vi "Main.vi"() -> ()   [LabVIEW 2017, in "Application.lvlib"]
doc: "This VI is the main application VI in the Delacor QMH project template. This application VI is implemented as a simple state machine, which communicates with two different Delacor QMH modules.\n_____\nBased on Delacor QMH Project Template 3.1.0.34."
uses:
  Application.lvlib
  Application Data--cluster.ctl
  State--enum.ctl
  GUI/GUI.lvlib
  Konfiguracja/Konfiguracja.lvlib
  Akwizycja/Akwizycja.lvlib
panel:
  in  "Debug":bool
  in  "Start Akwizycja Module":bool
  in  "Stop Akwizycja Module":bool caption="Start Akwizycja Module"
  out "Akwizycja Running?":bool
  out "version":string
  in  "Hide GUI Module":bool
  in  "Show GUI Module":bool
  in  "Stop GUI Module":bool
  in  "Start GUI Module":bool caption="Start Akwizycja Module"
  out "GUI Running?":bool
  in  "Hide Konfiguracja Module":bool
  in  "Show Konfiguracja Module":bool
  in  "Stop Konfiguracja Module":bool
  in  "Start Konfiguracja Module":bool
  out "Konfiguracja Running?":bool
  out "Status":string
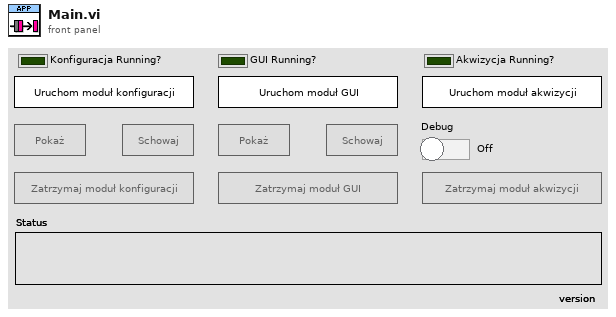
[diagram p1: front panel]
types:
  T1 = typedef "Application.lvlib/State--enum.ctl" = enum16{"Initialize", "Initialize Panel", "UI Interlocks", "Update Status", "Wait for Event", "Exit"}
  T2 = typedef "Application.lvlib/Application Data--cluster.ctl" = cluster{"Status":string, "Konfiguracja Controls":refnum<vi>[], "GUI Controls":refnum<vi>[], "Akwizycja Controls":refnum<vi>[]}
  T3 = typedef "Akwizycja.lvlib/Broadcast Events--cluster.ctl" = cluster{"Module Did Init":refnum<user-event>, "Status Updated":refnum<user-event>, "Error Reported":refnum<user-event>, "Module Did Stop":refnum<user-event>, "Update Module Execution Status":refnum<user-event>}
  T4 = typedef "GUI.lvlib/Broadcast Events--cluster.ctl" = cluster{"Module Did Init":refnum<user-event>, "Status Updated":refnum<user-event>, "Error Reported":refnum<user-event>, "Module Did Stop":refnum<user-event>, "Update Module Execution Status":refnum<user-event>, "Subpanel VI Loaded":refnum<user-event>}
  T5 = typedef "Konfiguracja.lvlib/Broadcast Events--cluster.ctl" = cluster{"Module Did Init":refnum<user-event>, "Status Updated":refnum<user-event>, "Error Reported":refnum<user-event>, "Module Did Stop":refnum<user-event>, "Update Module Execution Status":refnum<user-event>, "Subpanel VI Loaded":refnum<user-event>}
  T6 = enum8{"Enabled", "Disabled", "Disabled and Grayed Out"}
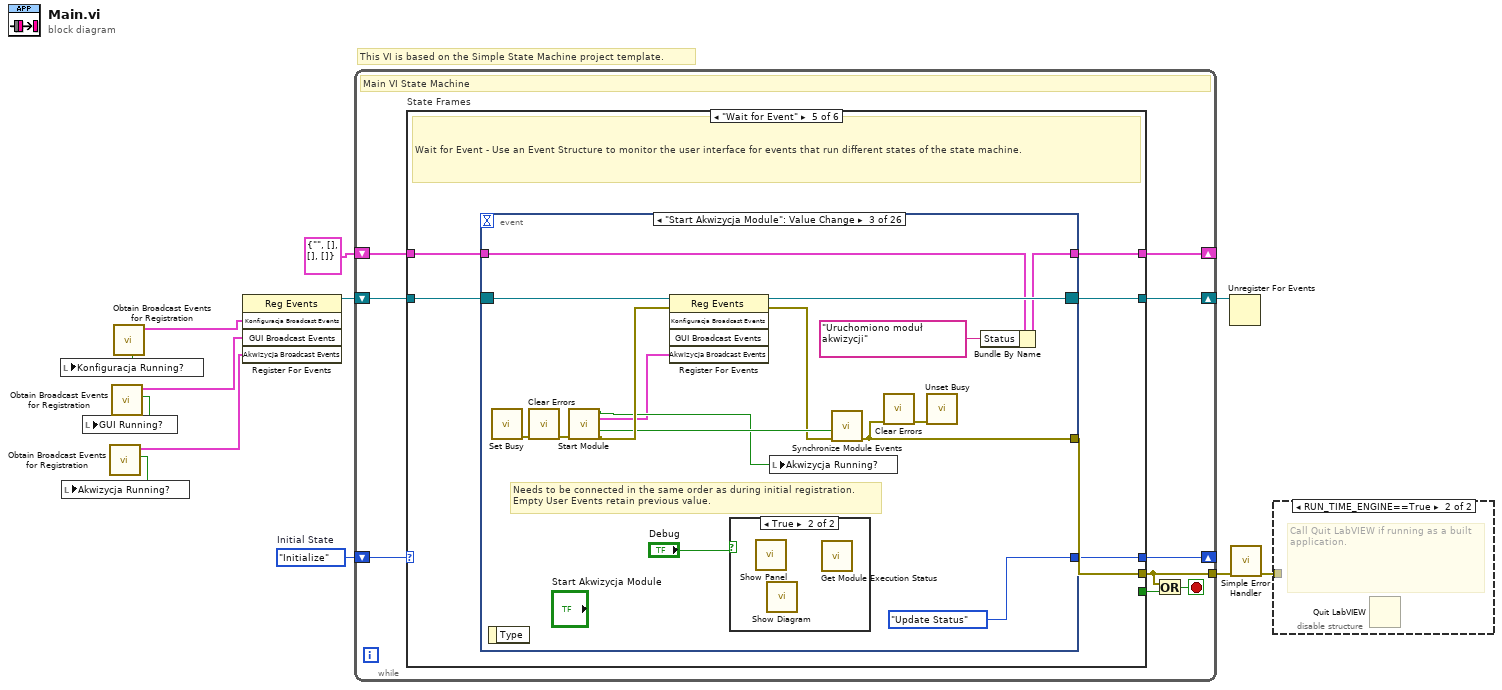
[diagram p0: block diagram]
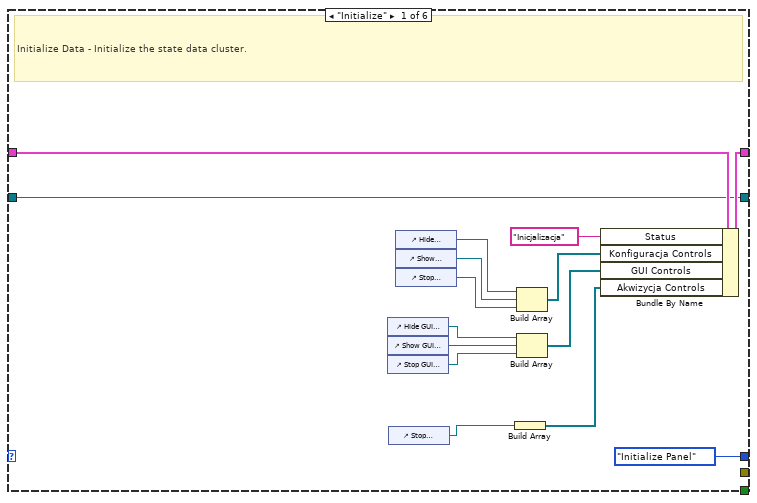
[diagram p2: hidden frame]
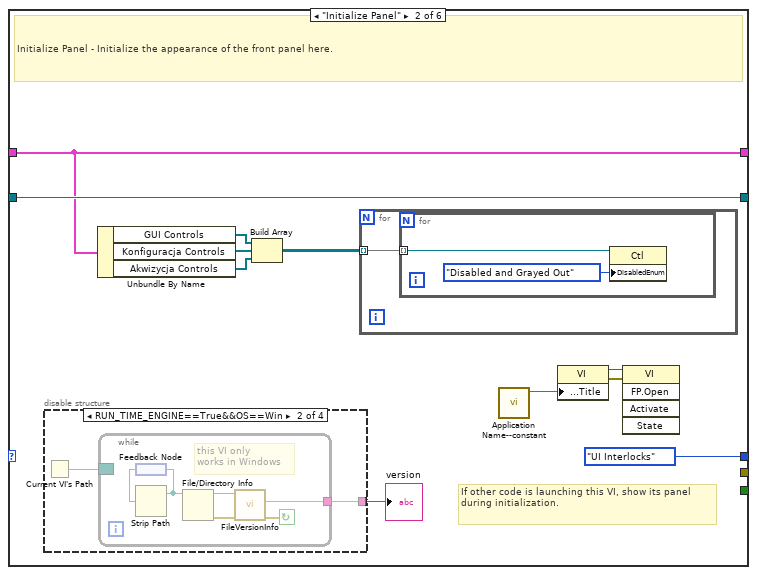
[diagram p3: hidden frame]
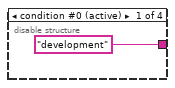
[diagram p4: hidden frame]
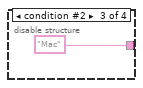
[diagram p5: hidden frame]
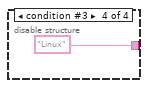
[diagram p6: hidden frame]
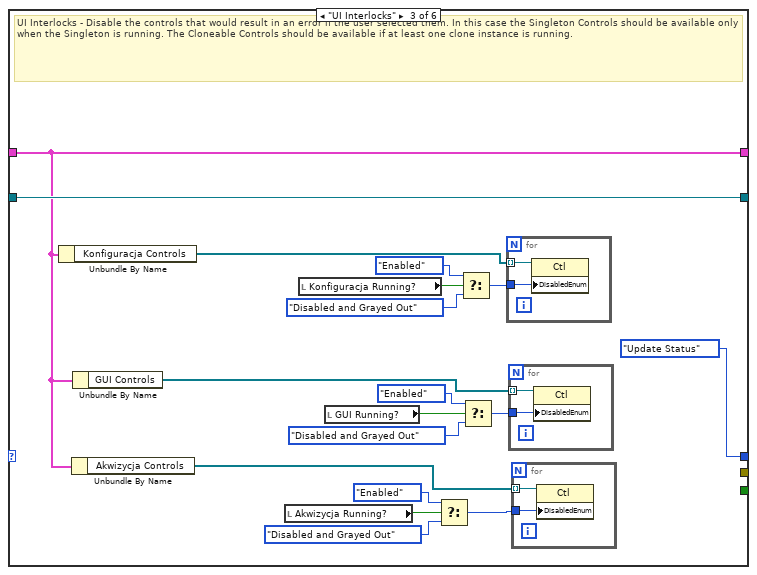
[diagram p7: hidden frame]
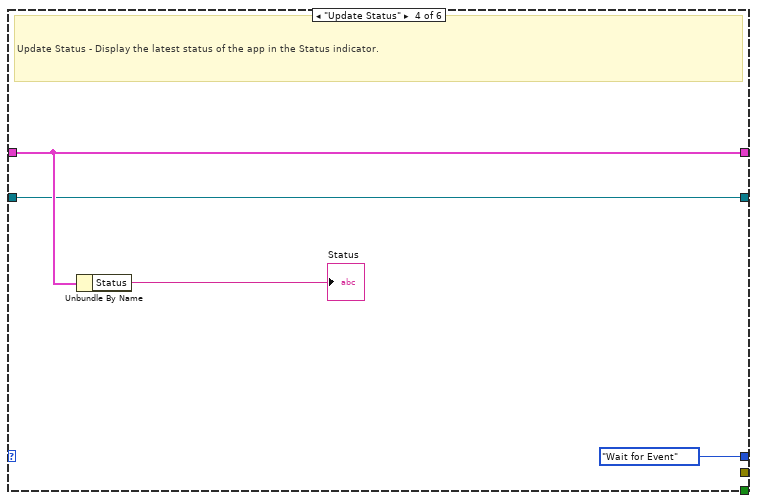
[diagram p8: hidden frame]
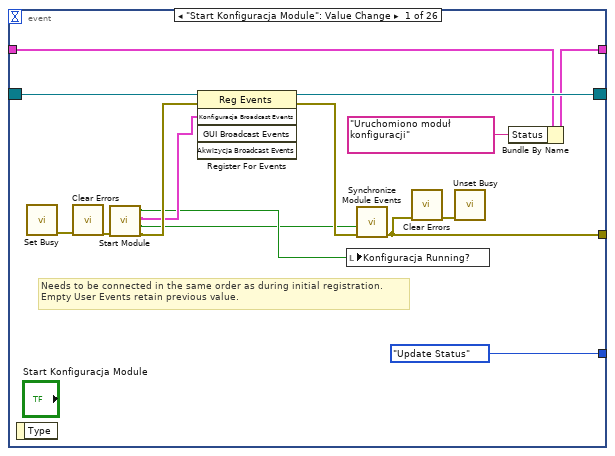
[diagram p9: hidden frame]
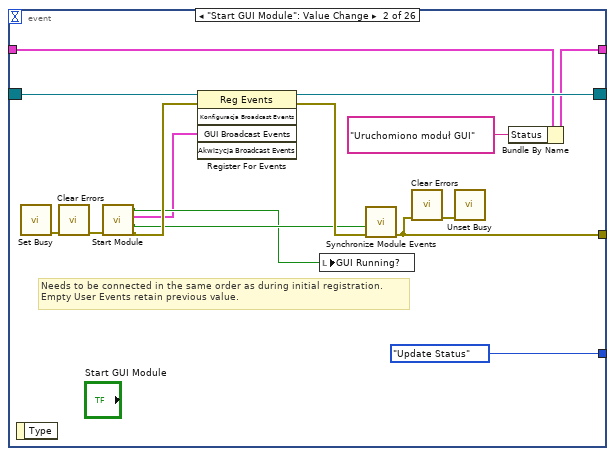
[diagram p10: hidden frame]
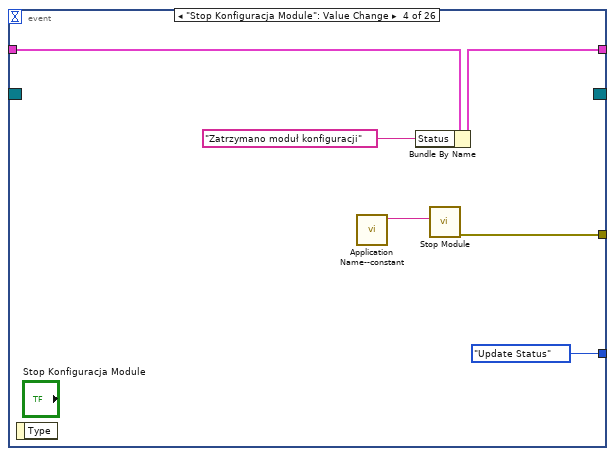
[diagram p12: hidden frame]
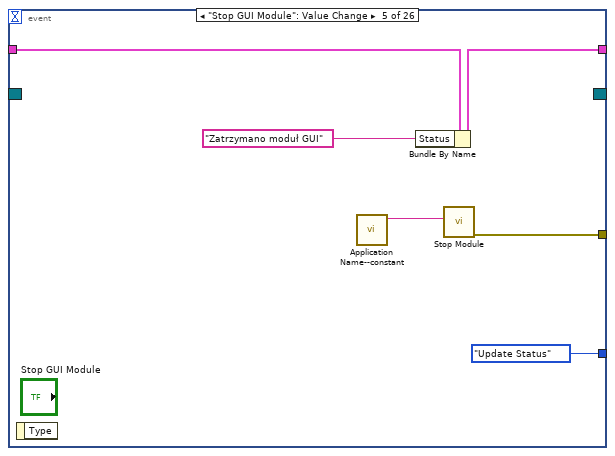
[diagram p13: hidden frame]
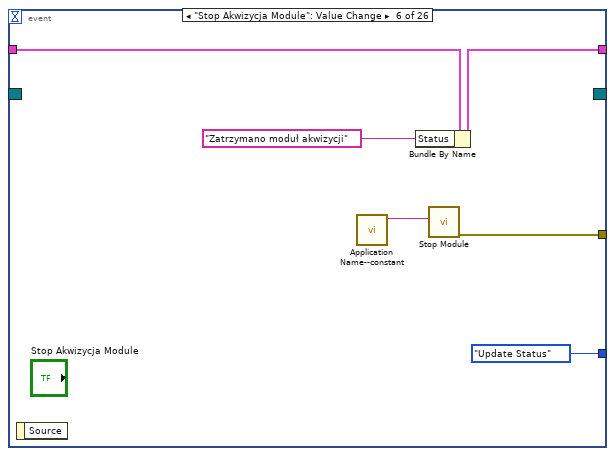
[diagram p14: hidden frame]
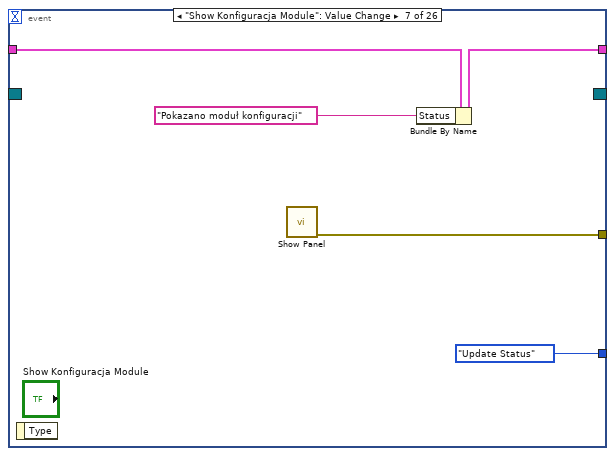
[diagram p15: hidden frame]
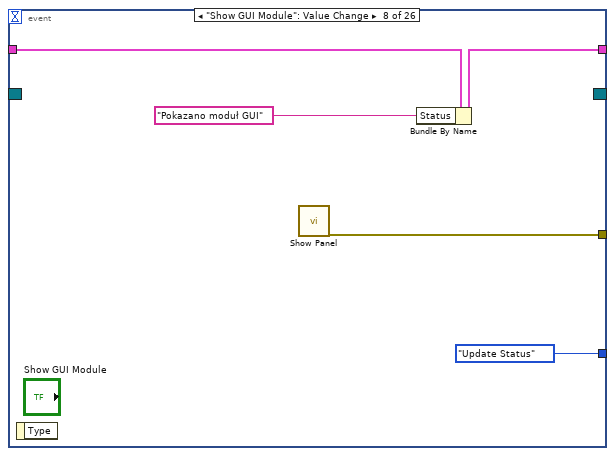
[diagram p16: hidden frame]
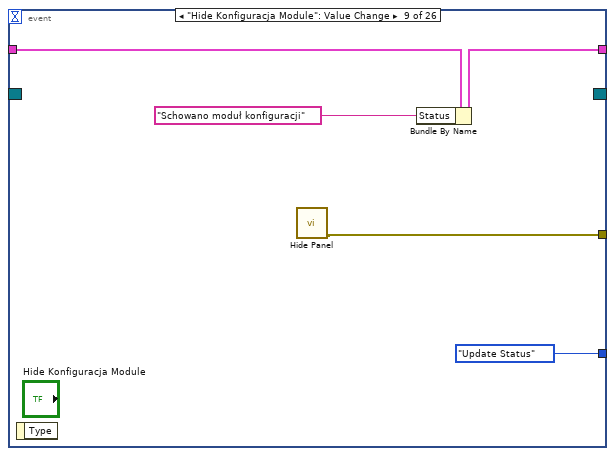
[diagram p17: hidden frame]
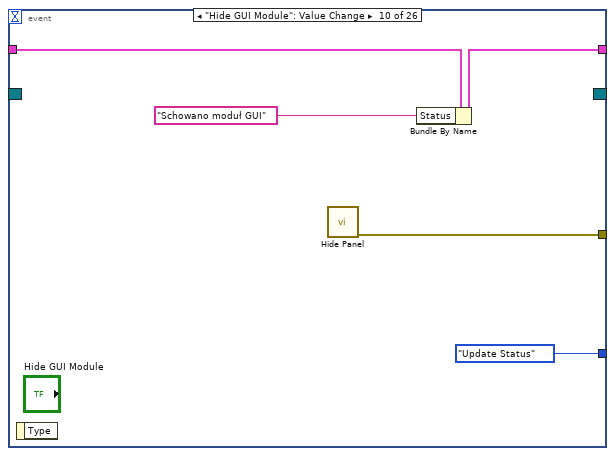
[diagram p18: hidden frame]
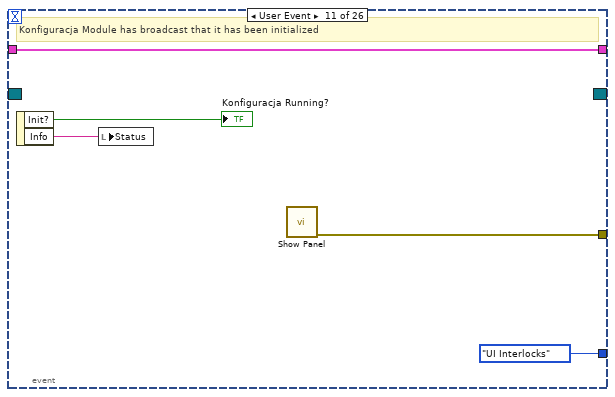
[diagram p19: hidden frame]
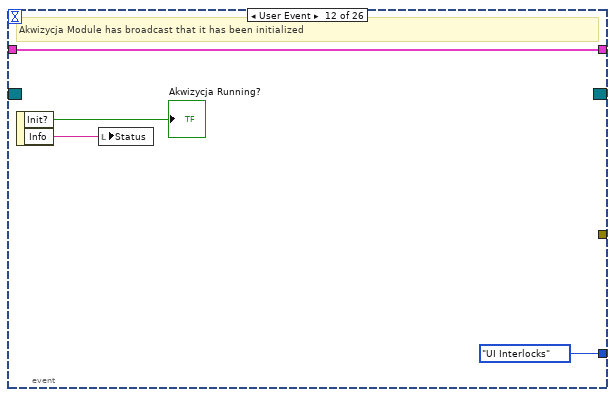
[diagram p20: hidden frame]
diagram:
  w9 = State--enum."Initialize"  # Initial State
  # "This VI is based on the Simple State Machine project template."
  n1 = call "Obtain Broadcast Events for Registration.vi"() -> ("Already running?"=w2:bool, "Akwizycja Broadcast Events"=w1:T3)  [unwired: 9 in, 1 out]
  n2 = local write "Akwizycja Running?"(w2) -> ()
  n3 = call "Obtain Broadcast Events for Registration.vi"() -> ("Already running?"=w5:bool, "GUI Broadcast Events"=w6:T4)  [unwired: 9 in, 1 out]
  n4 = local write "GUI Running?"(w5) -> ()
  n5 = call "Obtain Broadcast Events for Registration.vi"() -> ("Already running?"=w3:bool, "Konfiguracja Broadcast Events"=w4:T5)  [unwired: 9 in, 1 out]
  n6 = local write "Konfiguracja Running?"(w3) -> ()
  n7 = register-events(w4, w6, w1) -> (reference out=w8:refnum<event-registration>)  [unwired: 2 in, 1 out]
  n8 = while {
    shift-right: [w20] -> _
    shift-left: T2 {"Status"="", "Konfiguracja Controls"=[], "GUI Controls"=[], "Akwizycja Controls"=[]} ("Data Cluster") -> [w21]
    tunnel: [w16] -> w11
    shift-right: [w15] -> _
    shift-left: w9 -> [w18]
    shift-right: [w13] -> w7
    shift-left: w8 -> [w14]
    stop <- w17 stop-if-true
    # "Main VI State Machine"
    n9 = case "State Frames" shown="\"Wait for Event\"" w18 {
      tunnel: [_ _ _ _ w91 w275] -> w16
      tunnel: w21 -> [w36 w41 w67 w89 w93 w279]
      tunnel: [w35 w41 w67 w89 w92 w279] -> w20
      tunnel: [_ _ _ _ _ w278] -> w19
      tunnel: [State--enum."Initialize Panel" ("State") State--enum."UI Interlocks" ("State") State--enum."Update Status" ("State") State--enum."Wait for Event" ("State") w90 State--enum."Exit" ("State")] -> w15
      tunnel: w14 -> [w28 w46 w73 w86 w95 w276]
      tunnel: [w28 w46 w73 w86 w94 w276] -> w13
      frame "Initialize" {
        # "Initialize Data - Initialize the state data cluster."
        n10 = control-ref of="Hide GUI Module"() -> (w27:refnum<vi>)
        n11 = control-ref of="Show GUI Module"() -> (w26:refnum<vi>)
        n12 = control-ref of="Stop GUI Module"() -> (w25:refnum<vi>)
        n13 = control-ref of="Stop Akwizycja Module"() -> (w23:refnum<vi>)
        n14 = control-ref of="Hide Konfiguracja Module"() -> (w33:refnum<vi>)
        n15 = control-ref of="Show Konfiguracja Module"() -> (w32:refnum<vi>)
        n16 = control-ref of="Stop Konfiguracja Module"() -> (w31:refnum<vi>)
        n17 = Build Array(w23) -> (w22:refnum<vi>[])
        n18 = Build Array(w33, w32, w31) -> (w30:refnum<vi>[])
        n19 = Build Array(w27, w26, w25) -> (w24:refnum<vi>[])
        n20 = Bundle By Name(cluster=w36, "Status"="Inicjalizacja" ("Initial Message"), "Konfiguracja Controls"=w30, "GUI Controls"=w24, "Akwizycja Controls"=w22) -> (w35:T2)
      }
      frame "Initialize Panel" {
        # "If other code is launching this VI, show its panel during initialization."
        # "Initialize Panel - Initialize the appearance of the front panel here."
        n21 = disable-structure "Conditional Disable Structure" shown="RUN_TIME_ENGINE==True&&OS==Win" {
          disable-tunnel: ["development" w52 "Mac" "Linux"] -> w42
          frame condition #0 (active) {
          }
          frame condition #1 {
            n22 = Current VI's Path() -> (path=w53:path)
            n23 = while {
              border: w53 -> [_]
              tunnel: [w54] -> w52
              stop <- w55 continue-if-true
              # "this VI only \nworks in Windows"
              n24 = feedback #1() -> (w59:path)
              n25 = Strip Path(path=w59) -> (stripped path=w58:path)  [unwired: 1 out]
              n26 = feedback-in #1(w58) -> ()
              n27 = File/Directory Info(path=w58) -> (path out=w56:path, error out=w57:errorcluster)  [unwired: 1 in, 5 out]
              n28 = call <vilib>:"FileVersionInfo.vi"("error in (no error)"=w57, "Application Path in"=w56) -> ("error out"=w55:errorcluster, "File Version Info"=w54:string)  [unwired: 6 in, 2 out]
            }
          }
          frame condition #2 {
          }
          frame condition #3 {
          }
        }
        "version" <- w42
        n29 = Unbundle By Name(w41) -> ("GUI Controls"=w40:refnum<vi>[], "Konfiguracja Controls"=w39:refnum<vi>[], "Akwizycja Controls"=w38:refnum<vi>[])
        n30 = Build Array(w40, w39, w38) -> (w37:refnum<vi>[][])
        n31 = for {
          tunnel: w37 -> [w48] mode=indexing
          n32 = for {
            tunnel: w48 -> [w49] mode=indexing
            n33 = property on="Property Node" class="Ctl"(reference=w49, "DisabledEnum"=T6."Disabled and Grayed Out" ("Disabled")) -> ()  [unwired: 1 in, 2 out]
          }
        }
        n34 = call "Application Name--constant.vi"() -> ("Application Name"=w45:string)  [unwired: 11 in]
        n35 = property on="Property Node" class="VI"("Front Panel.Title"=w45) -> (reference out=w44:refnum<vi>, error out=w43:errorcluster)  [unwired: 2 in]
        n36 = invoke class="VI" method="FP.Open"(reference=w44, error in=w43) -> ()  [unwired: 3 in, 5 out]
      }
      frame "UI Interlocks" {
        # "UI Interlocks - Disable the controls that would result in an error if the user selected them. In this case the Singleton Controls should be available only when the Singleton is running. The Cloneable Controls should be available if at least one clone instance is running."
        n37 = Unbundle By Name(w67) -> ("Konfiguracja Controls"=w76:refnum<vi>[])
        n38 = Unbundle By Name(w67) -> ("Akwizycja Controls"=w63:refnum<vi>[])
        n39 = Unbundle By Name(w67) -> ("GUI Controls"=w68:refnum<vi>[])
        n40 = local read "Akwizycja Running?"() -> (w66:bool)
        n41 = local read "Konfiguracja Running?"() -> (w75:bool)
        n42 = local read "GUI Running?"() -> (w69:bool)
        n43 = Select(t=T6."Enabled" ("Disabled"), s=w66, f=T6."Disabled and Grayed Out" ("Disabled")) -> (s? t:f=w62:T6)
        n44 = Select(t=T6."Enabled" ("Disabled"), s=w75, f=T6."Disabled and Grayed Out" ("Disabled")) -> (s? t:f=w77:T6)
        n45 = Select(t=T6."Enabled" ("Disabled"), s=w69, f=T6."Disabled and Grayed Out" ("Disabled")) -> (s? t:f=w70:T6)
        n46 = for {
          tunnel: w76 -> [w85] mode=indexing
          tunnel: w77 -> [w84]
          n47 = property on="Property Node" class="Ctl"(reference=w85, "DisabledEnum"=w84) -> ()  [unwired: 1 in, 2 out]
        }
        n48 = for {
          tunnel: w68 -> [w83] mode=indexing
          tunnel: w70 -> [w82]
          n49 = property on="Property Node" class="Ctl"(reference=w83, "DisabledEnum"=w82) -> ()  [unwired: 1 in, 2 out]
        }
        n50 = for {
          tunnel: w63 -> [w81] mode=indexing
          tunnel: w62 -> [w80]
          n51 = property on="Property Node" class="Ctl"(reference=w81, "DisabledEnum"=w80) -> ()  [unwired: 1 in, 2 out]
        }
      }
      frame "Update Status" {
        # "Update Status - Display the latest status of the app in the Status indicator."
        n52 = Unbundle By Name(w89) -> ("Status"=→"Status":string)
      }
      frame "Wait for Event" {
        # "Wait for Event - Use an Event Structure to monitor the user interface for events that run different states of the state machine."
        n53 = event shown="[2] \"Start Akwizycja Module\": Value Change" {
          selector: w95 -> [w109 w124 w140 _ _ _ _ _ _ _ _ _ _ _ _ _ _ _ _ _ _ _ _ _ _ _]
          dyn-events: [w108 w123 w139 _ _ _ _ _ _ _ _ _ _ _ _ _ _ _ _ _ _ _ _ _ _ _] -> w94
          timeout: _ -> [_ _ _ _ _ _ _ _ _ _ _ _ _ _ _ _ _ _ _ _ _ _ _ _ _ _]
          tunnel: [w96 w116 w129 w143 w148 w155 w160 w165 w170 w175 w180 _ w189 w194 _ w201 _ _ _ _ _ _ _ _ _ _] -> w91
          tunnel: [w105 w120 w136 w145 w151 w157 w163 w168 w173 w178 w182 w187 w193 w197 w200 w204 w206 w210 w214 w225 w235 w245 w250 w257 w264 w269] -> w92
          tunnel: w93 -> [w106 w121 w137 w146 w152 w158 w164 w169 w174 w179 w182 w187 w193 w197 w200 w204 w207 w211 w215 w226 w236 w246 w251 w258 w265 w269]
          tunnel: [State--enum."Update Status" ("State") State--enum."Update Status" ("State") State--enum."Update Status" ("State") State--enum."Update Status" ("State") State--enum."Update Status" ("State") State--enum."Update Status" ("State") State--enum."Update Status" ("State") State--enum."Update Status" ("State") State--enum."Update Status" ("State") State--enum."Update Status" ("State") State--enum."UI Interlocks" ("State") State--enum."UI Interlocks" ("State") State--enum."UI Interlocks" ("State") State--enum."UI Interlocks" ("State") State--enum."UI Interlocks" ("State") State--enum."UI Interlocks" ("State") State--enum."Update Status" ("State") State--enum."Update Status" ("State") State--enum."Update Status" ("State") State--enum."Update Status" ("State") State--enum."Update Status" ("State") State--enum."Update Status" ("State") State--enum."UI Interlocks" ("State") State--enum."UI Interlocks" ("State") State--enum."UI Interlocks" ("State") State--enum."Exit" ("State")] -> w90
          event "Start Konfiguracja Module": Value Change {
            # "Needs to be connected in the same order as during initial registration.\nEmpty User Events retain previous value."
            n54 = event-data() -> ()  [unwired: 1 in, 1 out]
            n55 = call <vilib>:"Set Busy.vi"() -> ("error out"=w110:errorcluster)  [unwired: 10 in, 1 out]
            n56 = call <vilib>:"Clear Errors.vi"("error in (no error)"=w110) -> ("error out"=w99:errorcluster)  [unwired: 5 in, 1 out]
            n57 = call "Start Module.vi"("error in (no error)"=w99) -> ("error out"=w102:errorcluster, "Wait for Event Sync?"=w97:bool, "Konfiguracja Broadcast Events"=w101:T5, "Module Was Already Running?"=w100:bool)  [unwired: 7 in]
            n58 = register-events(reference=w109, error in=w102, w101) -> (reference out=w108:refnum<event-registration>, error out=w98:errorcluster)  [unwired: 2 in]
            n59 = local write "Konfiguracja Running?"(w100) -> ()
            n60 = call "Synchronize Module Events.vi"("error in (no error)"=w98, "Wait for Event Sync?"=w97) -> ("error out"=w96:errorcluster)  [unwired: 9 in]
            n61 = call <vilib>:"Clear Errors.vi"("error in (no error)"=w96) -> ("error out"=w103:errorcluster)  [unwired: 5 in, 1 out]
            n62 = call <vilib>:"Unset Busy.vi"("error in (no error)"=w103) -> ()  [unwired: 10 in, 1 out]
            n63 = Bundle By Name(cluster=w106, "Status"="Uruchomiono moduł konfiguracji") -> (w105:T2)
          }
          event "Start GUI Module": Value Change {
            # "Needs to be connected in the same order as during initial registration.\nEmpty User Events retain previous value."
            n64 = event-data() -> ()  [unwired: 1 in, 1 out]
            n65 = call <vilib>:"Set Busy.vi"() -> ("error out"=w125:errorcluster)  [unwired: 10 in, 1 out]
            n66 = call <vilib>:"Clear Errors.vi"("error in (no error)"=w125) -> ("error out"=w115:errorcluster)  [unwired: 5 in, 1 out]
            n67 = call "Start Module.vi"("error in (no error)"=w115) -> ("error out"=w114:errorcluster, "Wait for Event Sync?"=w113:bool, "GUI Broadcast Events"=w111:T4, "Module Was Already Running?"=w112:bool)  [unwired: 7 in]
            n68 = register-events(reference=w124, error in=w114, w111) -> (reference out=w123:refnum<event-registration>, error out=w117:errorcluster)  [unwired: 2 in]
            n69 = local write "GUI Running?"(w112) -> ()
            n70 = call "Synchronize Module Events.vi"("error in (no error)"=w117, "Wait for Event Sync?"=w113) -> ("error out"=w116:errorcluster)  [unwired: 9 in]
            n71 = call <vilib>:"Clear Errors.vi"("error in (no error)"=w116) -> ("error out"=w118:errorcluster)  [unwired: 5 in, 1 out]
            n72 = call <vilib>:"Unset Busy.vi"("error in (no error)"=w118) -> ()  [unwired: 10 in, 1 out]
            n73 = Bundle By Name(cluster=w121, "Status"="Uruchomiono moduł GUI") -> (w120:T2)
          }
          event "Start Akwizycja Module": Value Change {
            # "Needs to be connected in the same order as during initial registration.\nEmpty User Events retain previous value."
            n74 = event-data() -> ()  [unwired: 1 in, 1 out]
            n75 = call <vilib>:"Set Busy.vi"() -> ("error out"=w141:errorcluster)  [unwired: 10 in, 1 out]
            n76 = call <vilib>:"Clear Errors.vi"("error in (no error)"=w141) -> ("error out"=w133:errorcluster)  [unwired: 5 in, 1 out]
            n77 = call "Start Module.vi"("error in (no error)"=w133) -> ("Module Was Already Running?"=w128:bool, "Akwizycja Broadcast Events"=w127:T3, "Wait for Event Sync?"=w131:bool, "error out"=w132:errorcluster)  [unwired: 11 in]
            n78 = register-events(reference=w140, error in=w132, w127) -> (reference out=w139:refnum<event-registration>, error out=w130:errorcluster)  [unwired: 2 in]
            n79 = case shown="True" "Debug" {
              frame False {
              }
              frame True {
                n80 = call "Show Panel.vi"() -> ()  [unwired: 11 in, 1 out]
                n81 = call "Show Diagram.vi"() -> ()  [unwired: 11 in, 1 out]
                n82 = call "Get Module Execution Status.vi"() -> ()  [unwired: 11 in, 1 out]
              }
            }
            n83 = local write "Akwizycja Running?"(w128) -> ()
            n84 = call "Synchronize Module Events.vi"("error in (no error)"=w130, "Wait for Event Sync?"=w131) -> ("error out"=w129:errorcluster)  [unwired: 9 in]
            n85 = call <vilib>:"Clear Errors.vi"("error in (no error)"=w129) -> ("error out"=w134:errorcluster)  [unwired: 5 in, 1 out]
            n86 = call <vilib>:"Unset Busy.vi"("error in (no error)"=w134) -> ()  [unwired: 10 in, 1 out]
            n87 = Bundle By Name(cluster=w137, "Status"="Uruchomiono moduł akwizycji") -> (w136:T2)
          }
          event "Stop Konfiguracja Module": Value Change {
            n88 = event-data() -> ()  [unwired: 1 in, 1 out]
            n89 = call "Application Name--constant.vi"() -> ("Application Name"=w142:string)  [unwired: 11 in]
            n90 = Bundle By Name(cluster=w146, "Status"="Zatrzymano moduł konfiguracji" ("Message")) -> (w145:T2)
            n91 = call "Stop Module.vi"("Origin"=w142) -> ("error out"=w143:errorcluster)  [unwired: 10 in]
          }
          event "Stop GUI Module": Value Change {
            n92 = event-data() -> ()  [unwired: 1 in, 1 out]
            n93 = call "Application Name--constant.vi"() -> ("Application Name"=w149:string)  [unwired: 11 in]
            n94 = Bundle By Name(cluster=w152, "Status"="Zatrzymano moduł GUI" ("Message")) -> (w151:T2)
            n95 = call "Stop Module.vi"("Origin"=w149) -> ("error out"=w148:errorcluster)  [unwired: 10 in]
          }
          event "Stop Akwizycja Module": Value Change {
            n96 = event-data() -> ()  [unwired: 1 in, 1 out]
            n97 = call "Application Name--constant.vi"() -> ("Application Name"=w154:string)  [unwired: 11 in]
            n98 = Bundle By Name(cluster=w158, "Status"="Zatrzymano moduł akwizycji" ("Message")) -> (w157:T2)
            n99 = call "Stop Module.vi"("Origin"=w154) -> ("error out"=w155:errorcluster)  [unwired: 10 in]
          }
          event "Show Konfiguracja Module": Value Change {
            n100 = event-data() -> ()  [unwired: 1 in, 1 out]
            n101 = call "Show Panel.vi"() -> ("error out"=w160:errorcluster)  [unwired: 11 in]
            n102 = Bundle By Name(cluster=w164, "Status"="Pokazano moduł konfiguracji" ("Message")) -> (w163:T2)
          }
          event "Show GUI Module": Value Change {
            n103 = event-data() -> ()  [unwired: 1 in, 1 out]
            n104 = call "Show Panel.vi"() -> ("error out"=w165:errorcluster)  [unwired: 11 in]
            n105 = Bundle By Name(cluster=w169, "Status"="Pokazano moduł GUI" ("Message")) -> (w168:T2)
          }
          event "Hide Konfiguracja Module": Value Change {
            n106 = event-data() -> ()  [unwired: 1 in, 1 out]
            n107 = call "Hide Panel.vi"() -> ("error out"=w170:errorcluster)  [unwired: 11 in]
            n108 = Bundle By Name(cluster=w174, "Status"="Schowano moduł konfiguracji" ("Message")) -> (w173:T2)
          }
          event "Hide GUI Module": Value Change {
            n109 = event-data() -> ()  [unwired: 1 in, 1 out]
            n110 = call "Hide Panel.vi"() -> ("error out"=w175:errorcluster)  [unwired: 11 in]
            n111 = Bundle By Name(cluster=w179, "Status"="Schowano moduł GUI" ("Message")) -> (w178:T2)
          }
          event User Event {
            # "Konfiguracja Module has broadcast that it has been initialized"
            n112 = event-data() -> ("Init?"=→"Konfiguracja Running?":bool, "Info"=w184:string)  [unwired: 1 in]
            n113 = local write "Status"(w184) -> ()
            n114 = call "Show Panel.vi"() -> ("error out"=w180:errorcluster)  [unwired: 11 in]
          }
          event User Event {
            # "Akwizycja Module has broadcast that it has been initialized"
            n115 = event-data() -> ("Init?"=→"Akwizycja Running?":bool, "Info"=w188:string)  [unwired: 1 in]
            n116 = local write "Status"(w188) -> ()
          }
          event User Event {
            # "GUI Module has broadcast that it has been initialized"
            n117 = event-data() -> ("Init?"=→"GUI Running?":bool, "Info"=w191:string)  [unwired: 1 in]
            n118 = local write "Status"(w191) -> ()
            n119 = call "Show Panel.vi"() -> ("error out"=w189:errorcluster)  [unwired: 11 in]
          }
          event User Event {
            # "Konfiguracja Module has broadcast its execution status"
            n120 = event-data() -> ("Running?"=w195:bool)  [unwired: 1 in]
            n121 = local write "Konfiguracja Running?"(w195) -> ()
            n122 = call "Show Panel.vi"() -> ("error out"=w194:errorcluster)  [unwired: 11 in]
          }
          event User Event {
            # "Konfiguracja Module has broadcast its execution status"
            n123 = event-data() -> ("Running?"=w198:bool)  [unwired: 1 in]
            n124 = local write "Akwizycja Running?"(w198) -> ()
          }
          event User Event {
            # "GUI Module has broadcast its execution status"
            n125 = event-data() -> ("Running?"=w202:bool)  [unwired: 1 in, 1 out]
            n126 = local write "GUI Running?"(w202) -> ()
            n127 = call "Show Panel.vi"() -> ("error out"=w201:errorcluster)  [unwired: 11 in]
          }
          event User Event {
            # "Konfiguracja Module has broadcast its status"
            n128 = event-data() -> ("Status"=w208:string)  [unwired: 1 in]
            n129 = Bundle By Name(cluster=w207, "Status"=w208) -> (w206:T2)
          }
          event User Event {
            # "Akwizycja Module has broadcast its status"
            n130 = event-data() -> ("Status"=w212:string)  [unwired: 1 in]
            n131 = Bundle By Name(cluster=w211, "Status"=w212) -> (w210:T2)
          }
          event User Event {
            # "GUI Module has broadcast its status"
            n132 = event-data() -> ("Status"=w216:string)  [unwired: 1 in]
            n133 = Bundle By Name(cluster=w215, "Status"=w216) -> (w214:T2)
          }
          event User Event {
            # "Konfiguracja Module had an error"
            n134 = event-data() -> ("Module Name"=w218:string, "Additional Information"=w223:string, "Error"=w222:errorcluster)  [unwired: 1 in]
            n135 = Unbundle By Name(w222) -> ("code"=w217:i32, "source"=w221:string)
            n136 = Format Into String(format string="Error code %d Module: %s  Additional Information: %s\nSource: %s", w217, w218, w223, w221) -> (resulting string=w219:string)  [unwired: 2 in, 1 out]
            n137 = Bundle By Name(cluster=w226, "Status"=w219) -> (w225:T2)
          }
          event User Event {
            # "Akwizycja Module had an error"
            n138 = event-data() -> ("Module Name"=w228:string, "Additional Information"=w233:string, "Error"=w232:errorcluster)  [unwired: 1 in]
            n139 = Unbundle By Name(w232) -> ("code"=w227:i32, "source"=w231:string)
            n140 = Format Into String(format string="Error code %d Module: %s  Additional Information: %s\nSource: %s", w227, w228, w233, w231) -> (resulting string=w229:string)  [unwired: 2 in, 1 out]
            n141 = Bundle By Name(cluster=w236, "Status"=w229) -> (w235:T2)
          }
          event User Event {
            # "GUI Module had an error"
            n142 = event-data() -> ("Module Name"=w238:string, "Additional Information"=w243:string, "Error"=w242:errorcluster)  [unwired: 1 in]
            n143 = Unbundle By Name(w242) -> ("code"=w237:i32, "source"=w241:string)
            n144 = Format Into String(format string="Error code %d Module: %s  Additional Information: %s\nSource: %s", w237, w238, w243, w241) -> (resulting string=w239:string)  [unwired: 2 in, 1 out]
            n145 = Bundle By Name(cluster=w246, "Status"=w239) -> (w245:T2)
          }
          event User Event {
            n146 = event-data() -> ("Origin"=w248:string)  [unwired: 1 in]
            n147 = local write "Konfiguracja Running?"(FALSE ("My Singleton Module Init?")) -> ()
            n148 = Concatenate Strings(w248, " Did Stop.") -> (w247:string)
            n149 = Bundle By Name(cluster=w251, "Status"=w247) -> (w250:T2)
          }
          event User Event {
            n150 = event-data() -> ("Origin"=w255:string)  [unwired: 1 in]
            n151 = local write "Akwizycja Running?"(FALSE ("My Singleton Module Init?")) -> ()
            n152 = Concatenate Strings(w255, " Did Stop.") -> (w254:string)
            n153 = Bundle By Name(cluster=w258, "Status"=w254) -> (w257:T2)
          }
          event User Event {
            n154 = event-data() -> ("Origin"=w262:string)  [unwired: 1 in]
            n155 = local write "GUI Running?"(FALSE ("My Singleton Module Init?")) -> ()
            n156 = Concatenate Strings(w262, " Did Stop.") -> (w261:string)
            n157 = Bundle By Name(cluster=w265, "Status"=w261) -> (w264:T2)
          }
          event Panel Close? {
            # "Go to the 'Exit' state if the user tries to close the panel."
            n158 = event-data() -> ()  [unwired: 1 in, 1 out]
            n159 = event-data ("Event Filter Node")("Discard?"=TRUE) -> ()  [unwired: 1 in, 1 out]
          }
        }
      }
      frame "Exit" {
        w272 = TRUE  # Wait for Module to stop?
        w278 = TRUE  # Stop the VI
        # "Zatrzymuje moduł konfiguracji i interfejs graficzny.\n\nNie zatrzymuje modułu akwizycji"
        # "Exit - Exit the application."
        n160 = call "Application Name--constant.vi"() -> ("Application Name"=w273:string)  [unwired: 11 in]
        n161 = call "Stop Module.vi"("Wait for Module to Stop? (F)"=w272, "Origin"=w273) -> ("error out"=w271:errorcluster)  [unwired: 9 in]
        n162 = call "Stop Module.vi"("Wait for Module to Stop? (F)"=w272, "Origin"=w273) -> ("error out"=w274:errorcluster)  [unwired: 9 in]
        n163 = Merge Errors(w271, w274) -> (w275:errorcluster)
      }
    }
    n164 = Or(x=w16, y=w19) -> (x .or. y?=w17:bool)
  }
  n165 = Unregister For Events(event registration refnum=w7) -> ()  [unwired: 1 in, 1 out]
  n166 = call <vilib>:"Simple Error Handler.vi"("error in (no error)"=w11) -> ("error out"=w10:errorcluster)  [unwired: 4 in, 4 out]
  n167 = disable-structure "Conditional Disable Structure" shown="RUN_TIME_ENGINE==True" {
    disable-tunnel: w10 -> [_ _]
    frame condition #0 (active) {
    }
    frame condition #1 {
      # "Call Quit LabVIEW if running as a built application."
      n168 = Quit LabVIEW() -> ()  [unwired: 1 in]
    }
  }
